vi "Initialize with Topology (Override Switches).vi"(7 "switches json":string, 8 "error in (no error)":errorcluster, 9 "reset device":bool=TRUE, 10 "topology":string, 11 "device":refnum<k21>) -> (0 "error out":errorcluster, 3 "session out":T1)   [LabVIEW 2020, in "SLSC Switch.lvlib"]
doc: "Returns a session handle used to identify the SLSC module in all subsequent SLSC Switch driver calls and sets the topology of the switch module."
uses:
  <vilib>/SLSC_Switch/SLSC Switch.lvlib
  nislscsl.dll
  <vilib>/userdefined/High Color/SLSC_Switch/nislscslSession.ctl
panel:
  in  "session in":T1
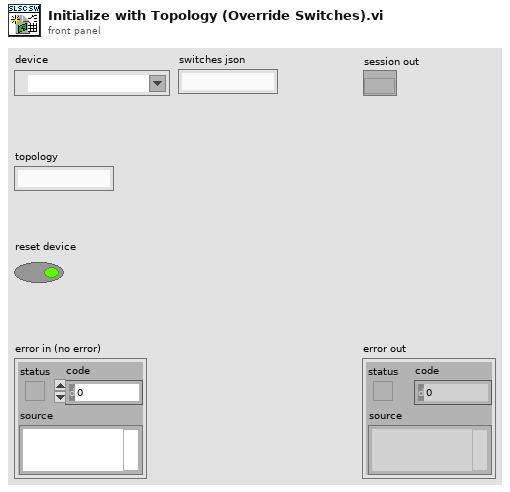
[diagram p1: front panel]
types:
  T1 = typedef "nislscslSession.ctl" = refnum<k20>
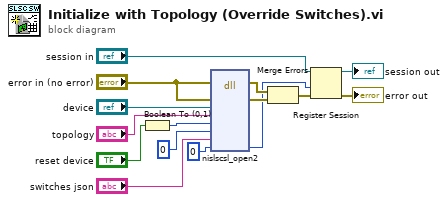
[diagram p0: block diagram]
diagram:
  n1 = Boolean To (0,1)(Boolean="reset device") -> (0, 1=w4:i16)
  n2 = dll-call lib="nislscsl.*" fn="nislscsl_open2"(error in="error in (no error)", "errorCluster"="error in (no error)", "deviceIdentifier"="device", "topologyName"="topology", "reset"=w4, "simulate"=u8 0, "capabilities"="switches json", "sessionHandlePtr"=u64 0) -> (error out=w12:errorcluster, "errorCluster"=w11:errorcluster, "sessionHandlePtr"=w10:u64)  [unwired: 8 in, 1 out]
  n3 = Merge Errors(w12, w11) -> (w9:errorcluster)
  n4 = Register Session(8:w9, 9:w10, 11:"session in") -> (0:→"error out":errorcluster, 3:→"session out":T1)  [unwired: 2 in]
